vi "Subvi_Online_SVM_SWLDA_분석기_woF4.vi"(0 "rate":dbl=500.0 caption="Rate" format="%0.2f", 1 "samples per channel":i32=25, 4 "Brain_data_source":dbl[][](array[numeric]) caption="EEG_Raw_Data" format="%0.3f", 5 "Target_Flash_Order":i64[][](array[numeric]), 6 "Value":T1, 7 "svm_model_file":string, 8 "Matrix":T1, 10 "Target":path, 12 "Nontarget":path) -> (13 "EPR_발생_total":i16[](array[numeric]), 14 "output-0~8":i32, 15 "decision":dbl[](array[numeric]), 18 "SWLDA":dbl[](array[numeric]), 19 "ERP_Parameters":dbl[][](array[numeric]))   [LabVIEW 2014]
uses:
  <vilib>/Analysis/Matrix/Datatypes/RealMatrix.ctl
  <vilib>/Analysis/3filter.llb/Filter Passband Type.ctl
  <vilib>/Analysis/baseanly.llb/Mean (DBL).vi
  <vilib>/Analysis/3filter.llb/Butterworth Filter (DBL).vi
  <vilib>/Utility/file.llb/Read From Spreadsheet File (DBL).vi
  Subvi/Control_Panel.vi
  <vilib>/Analysis/Matrix/Numeric/Conversions/Array To Matrix - RA.vi
  <vilib>/Analysis/Matrix/Numeric/Multiply/Multiply - RM,RM.vi
  <vilib>/Analysis/Matrix/Numeric/Subtract/Subtract - RM,RM.vi
  <vilib>/Analysis/Matrix/Numeric/Conversions/Matrix To Array - RM.vi
  <vilib>/Analysis/NI_AALBase.lvlib
  <vilib>/Analysis/Matrix/NI_Matrix.lvlib
  <vilib>/Analysis/Matrix/Numeric/Conversions/Array To Matrix - RA2.vi
panel:
  out "Real":dbl
  out "deleted portion":dbl[][](array[numeric])
  out "2-D Array of Real 3":dbl[][](array[numeric])
  out "2-D Array of Real 2":dbl[][](array[numeric])
  out "2-D Array of Real":dbl[][](array[numeric])
  out "1-D Array of Real":dbl[](array[numeric])
  out "SWLDA_original":dbl[][](array[numeric])
  out "size(s)":i32[](array[numeric])
  in  "LDA":path=path "C:/Users/Administrator/Desktop/공공복지안전사업연구-노수진/파일럿20130902/LDA_Matrix_Value.xls"
  out "전치된 배열":dbl[][](array[numeric])
  out "#channel":i32
  out "#sti 6":i32
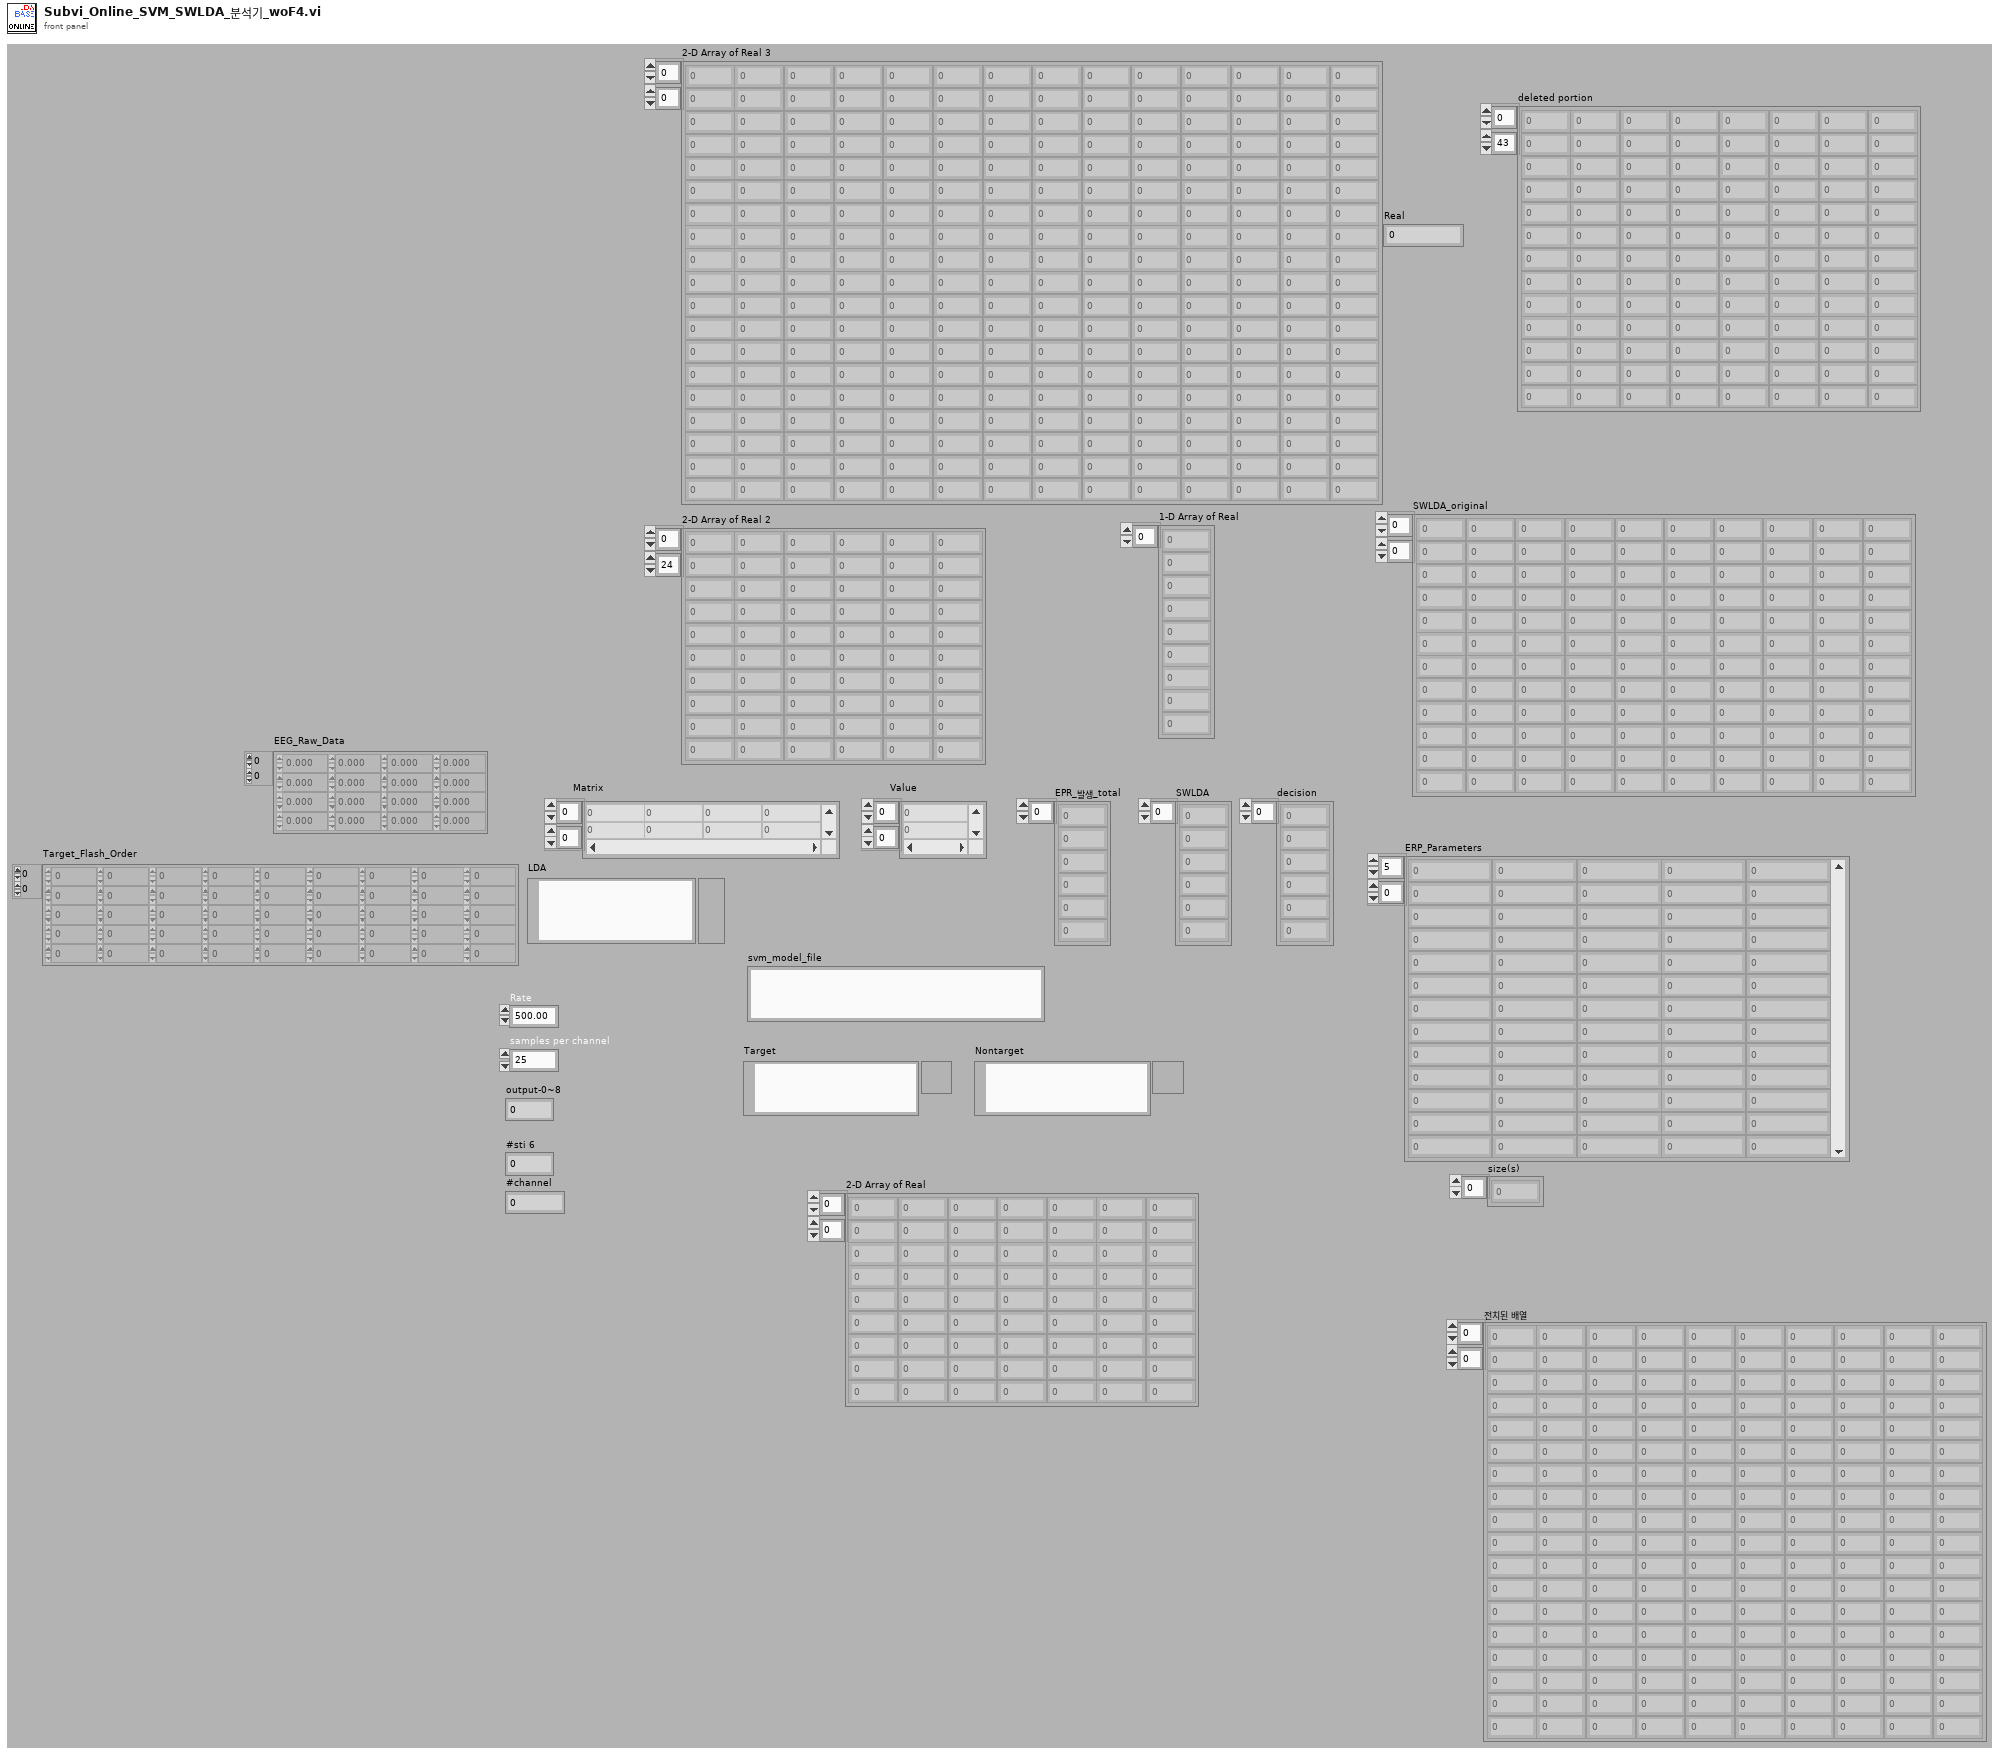
[diagram p1: front panel]
types:
  T1 = typedef "NI_Matrix.lvlib/RealMatrix.ctl" = dbl[][]
  T2 = typedef "NI_AALBase.lvlib/Filter Passband Type.ctl" = enum32{"Lowpass", "Highpass", "Bandpass", "Bandstop"}
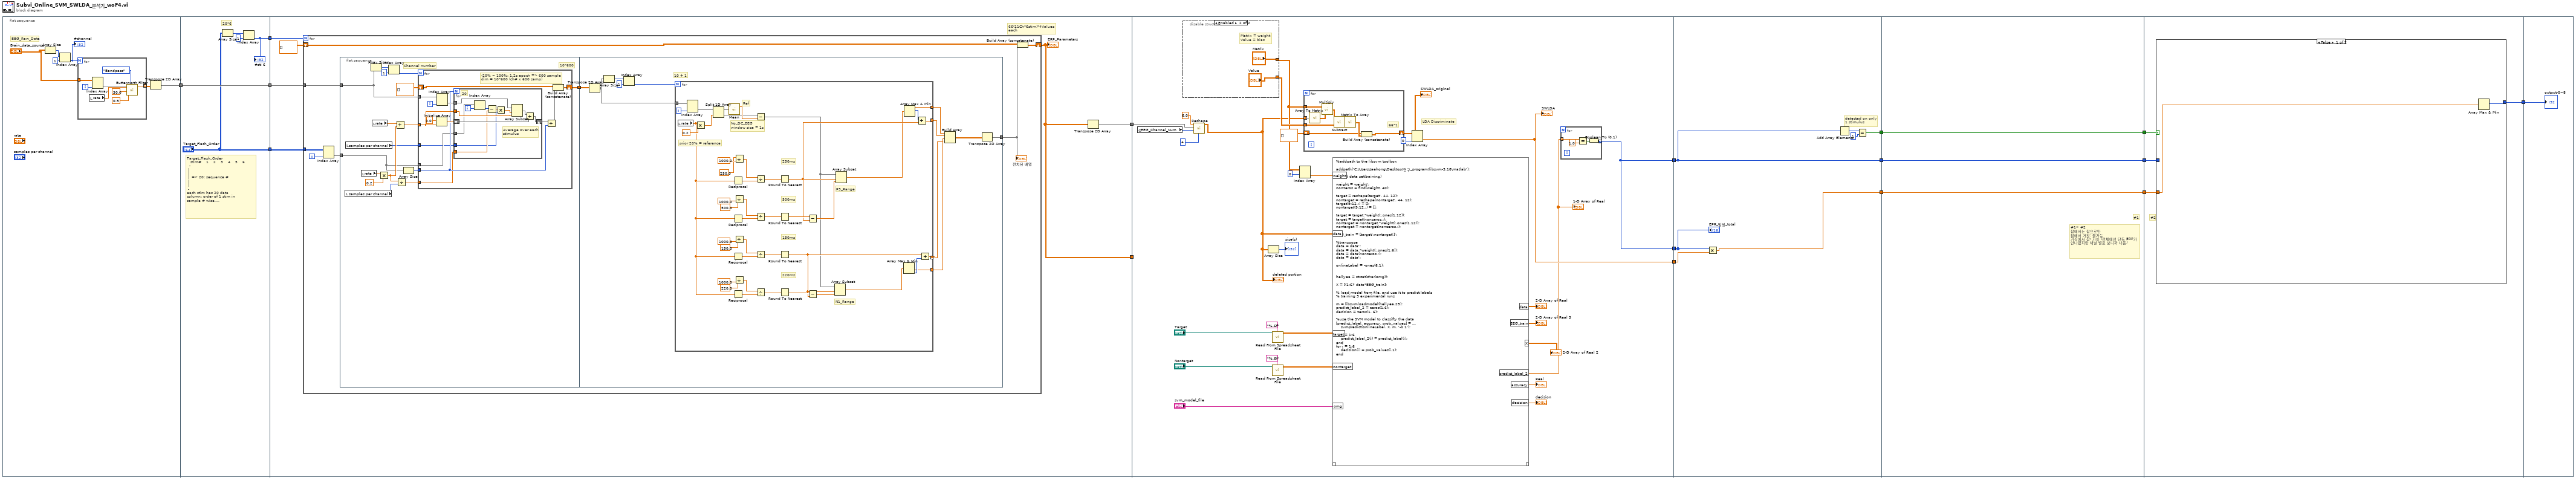
[diagram p0: block diagram]
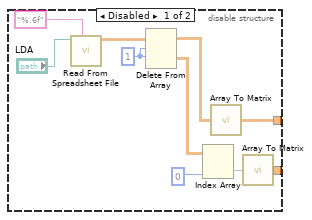
[diagram p2: hidden frame]
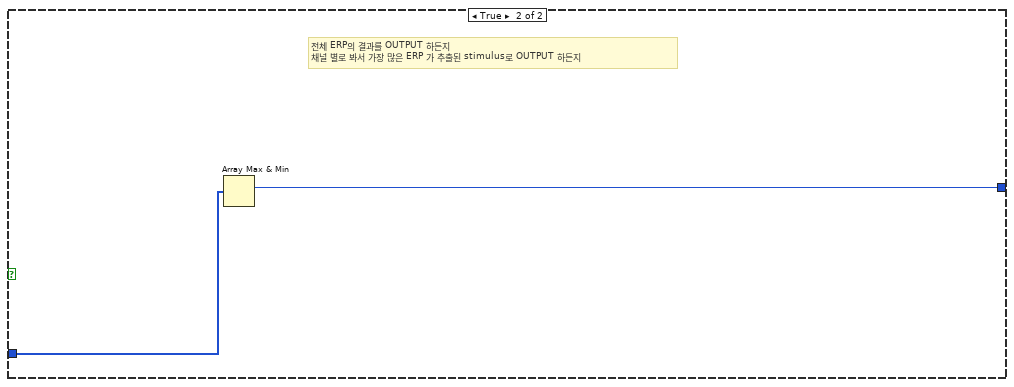
[diagram p3: hidden frame]
diagram:
  n1 = flat-sequence {
    tunnel: [w18] -> w16
    tunnel: [w35] -> w15
    tunnel: ["Target_Flash_Order"] -> w14
    tunnel: w16 -> [w35]
    tunnel: [w32] -> w13
    tunnel: w15 -> [w41]
    tunnel: w14 -> [w40]
    tunnel: w13 -> [w39]
    tunnel: [w36] -> w12
    tunnel: [w37] -> w11
    tunnel: w12 -> [w155]
    tunnel: w11 -> [_]
    tunnel: [w171] -> w10
    tunnel: [w171] -> w8
    tunnel: [w167] -> w4
    tunnel: w10 -> [w200]
    tunnel: [w204] -> w9
    tunnel: w8 -> [w203]
    tunnel: [w201] -> w5
    tunnel: w4 -> [w202]
    tunnel: [w200] -> w3
    tunnel: w9 -> [w207]
    tunnel: [w209] -> w6
    tunnel: w5 -> [w209]
    tunnel: w3 -> [w208]
    tunnel: [w208] -> w2
    tunnel: [w207] -> w1
    tunnel: [w213] -> w7
    tunnel: w6 -> [w212]
    tunnel: w2 -> [w210]
    tunnel: w1 -> [w211]
    tunnel: w7 -> [w218]
    frame #0 {
      # "EEG_Raw_Data"
      n2 = Array Size(array="Brain_data_source") -> (size(s)=w19:i32[])
      n3 = Index Array(array=w19, index=1) -> (element=w21:i32)
      "#channel" <- w21
      n4 = for {
        N: w21 -> [_]
        tunnel: "Brain_data_source" -> [w30]
        tunnel: [w26] -> w22 mode=indexing
        i -> [w29]
        n5 = local read "rate"() -> (w23:dbl)
        n6 = Index Array(array=w30, index (col)=w29) -> (element=w28:dbl[])  [unwired: 1 in]
        n7 = call-poly <vilib>:"Butterworth Filter.vi"("filter type"=Filter_Passband_Type."Bandpass", "low cutoff freq: fl"=0.5, "high cutoff freq: fh"=30.0, "sampling freq: fs"=w23, "X"=w28) -> ("Filtered X"=w26:dbl[])  [unwired: 3 in, 1 out]
      }
      n8 = Transpose 2D Array(2D array=w22) -> (transposed array=w18:dbl[][])
    }
    frame #1 {
      # "Target_Flash_Order\n   stim#    1    2    3    4    5    6    \n  -\n |\n |\n |  => 20: sequence # \n |\n |\n -\neach stim has 20 data\ncolumn: order of 1 stim in \nsample # wise...."
      # "20*6"
      n9 = Array Size(array="Target_Flash_Order") -> (size(s)=w34:i32[])
      n10 = Index Array(array=w34, index=1 ("인덱스")) -> (element=w32:i32)
      "#sti 6" <- w32
    }
    frame #2 {
      # "66(11Ch*6stim)*4Values\neach"
      n11 = for {
        N: w39 -> [_]
        tunnel: w41 -> [w48]
        tunnel: w40 -> [w47]
        shift-right: [w44] -> w37
        shift-left: dbl[][] [] -> [w43]
        i -> [w46]
        n12 = Index Array(array=w47, index (col)=w46) -> (element=w45:i64[])  [unwired: 1 in]
        n13 = flat-sequence {
          tunnel: w48 -> [w52]
          tunnel: w45 -> [w51]
          tunnel: [w50] -> w49
          tunnel: w49 -> [w96]
          tunnel: [w92] -> w42
          frame #0 {
            # "10*600"
            # "Channel number"
            n14 = local read "samples per channel"() -> (w59:i32)
            n15 = local read "samples per channel"() -> (w58:i32)
            n16 = local read "rate"() -> (w61:dbl)
            n17 = Array Size(array=w52) -> (size(s)=w55:i32[])
            n18 = local read "rate"() -> (w63:dbl)
            n19 = Multiply(x=w61, y=0.2) -> (x*y=w65:dbl)
            n20 = Index Array(array=w55, index=1) -> (element=w57:i32)
            n21 = Add(x=w63, y=w65) -> (x+y=w64:dbl)
            n22 = Divide(x=w65, y=w59) -> (x/y=w62:dbl)
            n23 = Array Size(array=w51) -> (size(s)=w54:i32)
            n24 = for {
              N: w57 -> [_]
              tunnel: w58 -> [w66]
              tunnel: w64 -> [w77]
              shift-right: [w70] -> w50
              shift-left: dbl[][] [] -> [w72]
              tunnel: w54 -> [w71]
              tunnel: w52 -> [w69]
              tunnel: w51 -> [w68]
              tunnel: w62 -> [w67]
              i -> [w79]
              # "-20% ~ 100%: 1.2s epoch => 600 sample\ndim = 10*600 (ch# x 600 samp)"
              n25 = Initialize Array(0.0 ("element"), w77) -> (w76:dbl[])
              n26 = Index Array(array=w69, index (col)=w79) -> (element=w78:dbl[])  [unwired: 1 in]
              n27 = for {
                N: w71 -> [_]
                tunnel: w78 -> [w91]
                shift-right: [w88] -> w74
                shift-left: w76 -> [w89]
                tunnel: w77 -> [w87]
                tunnel: w68 -> [w85]
                tunnel: w67 -> [w83]
                tunnel: w66 -> [w81]
                i -> [w86]
                # "Average over each\nstimulus"
                # "20"
                n28 = Index Array(array=w85, index=w86) -> (element=w84:i64)
                n29 = Subtract(x=w84, y=w83) -> (x-y=w82:dbl)
                n30 = Multiply(x=w82, y=w81) -> (x*y=w80:dbl)
                n31 = Array Subset(array=w91, index=w80, length=w87) -> (w90:dbl[])
                n32 = Add(x=w90, y=w89) -> (x+y=w88:dbl[])
              }
              n33 = Divide(x=w74, y=w71) -> (x/y=w73:dbl[])
              n34 = Build Array (concatenate)(w72, w73) -> (w70:dbl[][])
            }
          }
          frame #1 {
            # "10 + 1"
            n35 = Transpose 2D Array(2D array=w96) -> (transposed array=w94:dbl[][])
            n36 = Array Size(array=w94) -> (size(s)=w97:i32[])
            n37 = Index Array(array=w97, index=1) -> (element=w93:i32)
            n38 = for {
              N: w93 -> [_]
              tunnel: w94 -> [w146]
              tunnel: [w141] -> w101 mode=indexing
              tunnel: [w139] -> w100 mode=indexing
              tunnel: [w110] -> w99 mode=indexing
              tunnel: [w136] -> w98 mode=indexing
              i -> [w135]
              # "P3_Range"
              # "N1_Range"
              # "220ms"
              # "150ms"
              # "500ms"
              # "250ms"
              # "No_DC_EEG\nwindow size = 1s"
              # "Ref"
              # "prior 20% = reference"
              n39 = local read "rate"() -> (w117:dbl)
              n40 = Index Array(array=w146, index (col)=w135) -> (element=w138:dbl[])  [unwired: 1 in]
              n41 = Multiply(x=w117, y=0.2) -> (x*y=w144:dbl)
              n42 = Split 1D Array(array=w138, index=w144) -> (first subarray=w143:dbl[], second subarray=w134:dbl[])
              n43 = call-poly <vilib>:"Mean.vi"("X"=w143) -> ("mean"=w142:dbl)  [unwired: 1 out]
              n44 = Reciprocal(x=w117) -> (1/x=w133:dbl)
              n45 = Reciprocal(x=w117) -> (1/x=w132:dbl)
              n46 = Reciprocal(x=w117) -> (1/x=w131:dbl)
              n47 = Reciprocal(x=w117) -> (1/x=w130:dbl)
              n48 = Divide(x=250.0, y=1000.0) -> (x/y=w129:dbl)
              n49 = Divide(x=500.0, y=1000.0) -> (x/y=w128:dbl)
              n50 = Divide(x=150.0, y=1000.0) -> (x/y=w127:dbl)
              n51 = Divide(x=220.0, y=1000.0) -> (x/y=w126:dbl)
              n52 = Subtract(x=w134, y=w142) -> (x-y=w103:dbl[])
              n53 = Divide(x=w129, y=w133) -> (x/y=w116:dbl)
              n54 = Divide(x=w128, y=w132) -> (x/y=w115:dbl)
              n55 = Divide(x=w127, y=w131) -> (x/y=w114:dbl)
              n56 = Divide(x=w126, y=w130) -> (x/y=w113:dbl)
              n57 = Round To Nearest(number=w116) -> (nearest integer value=w106:dbl)
              n58 = Round To Nearest(number=w115) -> (nearest integer value=w112:dbl)
              n59 = Round To Nearest(number=w114) -> (nearest integer value=w108:dbl)
              n60 = Round To Nearest(number=w113) -> (nearest integer value=w111:dbl)
              n61 = Subtract(x=w112, y=w106) -> (x-y=w107:dbl)
              n62 = Subtract(x=w111, y=w108) -> (x-y=w109:dbl)
              n63 = Array Subset(array=w103, index=w108, length=w109) -> (w104:dbl[])
              n64 = Array Subset(array=w103, index=w106, length=w107) -> (w105:dbl[])
              n65 = Array Max & Min(array=w104) -> (min value=w110:dbl, min index (indices)=w137:i32)  [unwired: 2 out]
              n66 = Array Max & Min(array=w105) -> (max value=w141:dbl, max index (indices)=w140:i32)  [unwired: 2 out]
              n67 = Add(x=w140, y=w106) -> (x+y=w139:dbl)
              n68 = Add(x=w108, y=w137) -> (x+y=w136:dbl)
            }
            n69 = Build Array(w101, w100, w99, w98) -> (w95:dbl[][])
            n70 = Transpose 2D Array(2D array=w95) -> (transposed array=w92:dbl[][])
          }
        }
        n71 = Build Array (concatenate)(w43, w42) -> (w44:dbl[][])
        "전치된 배열" <- w42
      }
      "ERP_Parameters" <- w37
      n72 = Transpose 2D Array(2D array=w37) -> (transposed array=w36:dbl[][])
    }
    frame #3 {
      # "LDA Discriminate"
      # "66*1"
      n73 = global read "Control_Panel.vi" "EEG_Channel_Num"() -> (w154:i32)
      n74 = disable-structure shown="Enabled" {
        disable-tunnel: [w179 "Matrix"] -> w169
        disable-tunnel: [w178 "Value"] -> w170
        frame Disabled {
          w181 = 1 ("인덱스 (행)")
          n75 = call-poly <vilib>:"Read From Spreadsheet File.vi"("format (%.3f)"="%.6f", "file path (dialog if empty)"="LDA") -> ("all rows"=w175:dbl[][])  [unwired: 5 in, 4 out]
          n76 = Delete From Array(array=w175, length=w181, index (row)=w181) -> (deleted portion=w184:dbl[][], array with subset deleted=w183:dbl[][])  [unwired: 1 in]
          n77 = Index Array(array=w184, index (col)=0 ("인덱스")) -> (element=w182:dbl[])  [unwired: 1 in]
          n78 = call-poly <vilib>:"Array To Matrix.vi"("Real 2D Array"=w183) -> ("Real Matrix"=w179:T1)
          n79 = call-poly <vilib>:"Array To Matrix.vi"("Real 1D Array"=w182) -> ("Real Matrix (Column Vector)"=w178:T1)
        }
        frame Enabled {
          # "Matrix = weight\nValue = bias"
        }
      }
      n80 = call "Reshape.vi"("Numeric"=4, "EEG_Channel_Num"=w154, "all rows"=w155, "Numeric 2"=6.0) -> ("Array"=w151:dbl[][])  [unwired: 7 in]
      "deleted portion" <- w151
      n81 = Array Size(array=w151) -> (size(s)=→"size(s)":i32[])
      n82 = call-poly <vilib>:"Read From Spreadsheet File.vi"("format (%.3f)"="%.6f", "file path (dialog if empty)"="Target") -> ("all rows"=w163:dbl[][])  [unwired: 5 in, 4 out]
      n83 = call-poly <vilib>:"Read From Spreadsheet File.vi"("format (%.3f)"="%.6f", "file path (dialog if empty)"="Nontarget") -> ("all rows"=w162:dbl[][])  [unwired: 5 in, 4 out]
      n84 = Index Array(array=w169, index (row)=0) -> (element=w166:dbl[])  [unwired: 1 in]
      n85 = for {
        tunnel: w169 -> [w191]
        tunnel: w170 -> [w197]
        shift-right: [w194] -> w172
        shift-left: dbl[][] [] -> [w193]
        tunnel: w151 -> [w192] mode=indexing
        n86 = call-poly <vilib>:"Array To Matrix.vi"("Real 1D Array"=w192) -> ("Real Matrix (Column Vector)"=w196:T1)
        n87 = call-poly <vilib>:"Multiply.vi"("Real Matrix B"=w196, "Real Matrix A"=w191) -> ("A * B"=w199:T1)
        n88 = call-poly <vilib>:"Subtract.vi"("Real Matrix B"=w197, "Real Matrix A"=w199) -> ("A - B"=w198:T1)
        n89 = call-poly <vilib>:"Matrix To Array.vi"("Real Matrix"=w198) -> ("Real 2D Array"=w195:dbl[][])
        n90 = Build Array (concatenate)(w193, w195) -> (w194:dbl[][])
      }
      "SWLDA_original" <- w172
      n91 = script code="%addpath to the libsvm toolbox\n\naddpath('C:\\Users\\Jaehong\\Desktop\\연구_program\\libsvm-3.18\\matlab');\n\n%read data set(training)\n\nweight = weight';\nnonzeros = find(weight, 40);\n\ntarget = reshape(target', 44, 12);\nnontarget = reshape(nontarget', 44, 12);\ntarget(9:12,:) = [];\nnontarget(9:12,:) = [];\n\ntarget = target.*weight(:,ones(1,12));\ntarget = target(nonzeros,:);\nnontarget = nontarget.*weight(:,ones(1,12));\nnontarget = nontarget(nonzeros,:);\n\nEEG_train = [target';nontarget']';\n\n%transpose\ndata = data';\ndata = data.*weight(:,ones(1,6));\ndata = data(nonzeros,:);\ndata = data';\n\nonlineLabel = -ones(6,1);\n\n\nhellyea = strcat(char(omg));\n\nX = [(1:6)' data*EEG_train];\n\n% load model from file, and use it to predict labels\n% training 3 experimental runs\n\nm = libsvmloadmodel(hellyea,25);\npredict_label_2 = zeros(1,6);\ndecision = zeros(1, 6);\n\n%use the SVM model to classifty the data\n[predict_label, accuracy, prob_values] = ...\n    svmpredict(onlineLabel, X, m, '-b 1');\n\nfor i = 1:6\n    predict_label_2(i) = predict_label(i);\nend\nfor i = 1:6\n    decision(i) = prob_values(i,1);\nend"("weight"=w166, "target"=w163, "nontarget"=w162, "data"=w151, "omg"="svm_model_file") -> ("predict_label_2"=w161:dbl[], "data"=→"2-D Array of Real":dbl[][], "EEG_train"=→"2-D Array of Real 3":dbl[][], "X"=→"2-D Array of Real 2":dbl[][], "accuracy"=→"Real":dbl, "decision"=→"decision":dbl[])  [unwired: 1 in, 1 out]
      "1-D Array of Real" <- w161
      n92 = Index Array(array=w172, index (col)=0 ("비활성화된 인덱스 (열)")) -> (element=w167:dbl[])  [unwired: 1 in]
      "SWLDA" <- w167
      n93 = for {
        tunnel: w161 -> [w190] mode=indexing
        tunnel: [w189] -> w171 mode=indexing
        n94 = Equal?(x=w190, y=1.0) -> (x = y?=w187:bool)
        n95 = Boolean To (0,1)(Boolean=w187) -> (0, 1=w189:i16)
      }
    }
    frame #4 {
      # "detected on only\n1 stimulus"
      n96 = Multiply(x=w203, y=w202) -> (x*y=w201:dbl[])
      n97 = Add Array Elements(numeric array=w200) -> (sum=w206:i16)
      n98 = Equal?(x=w206, y=i16 1) -> (x = y?=w204:bool)
      "EPR_발생_total" <- w203
    }
    frame #5 {
      # "#1> #2\n참에서는 참으로만\n참에서 거짓: 불가능\n거짓에서 참: 가능 (전체에선 단독 ERP가 안나왔지만 채널 별로 보니까 나옴)"
      # "#1"
    }
    frame #6 {
      # "#2"
      n99 = case shown="False" w211 {
        tunnel: [w215 w217] -> w213
        tunnel: w212 -> [w214 _]
        tunnel: w210 -> [_ w216]
        frame False {
          n100 = Array Max & Min(array=w214) -> (max index (indices)=w215:i32)  [unwired: 3 out]
        }
        frame True {
          # "전체 ERP의 결과를 OUTPUT 하든지\n채널 별로 봐서 가장 많은 ERP 가 추출된 stimulus로 OUTPUT 하든지"
          n101 = Array Max & Min(array=w216) -> (max index (indices)=w217:i32)  [unwired: 3 out]
        }
      }
    }
    frame #7 {
      "output-0~8" <- w218
    }
  }
